vi "MainRunExp.vi"() -> ()   [LabVIEW 2019, in "MotorPID.lvlib"]
uses:
  MotorPID.lvlib
  RunState.ctl
  KNRm_ReMi_OS5.lvlibp/KNRm_ReMi_Toolkit/IO/LowLevel/IO_Channel_DIO.ctl
  <vilib>/Platform/TimedLoop/XDataNode/timing_clust.ctl
  <vilib>/Platform/TimedLoop/XDataNode/nitl_modes.ctl
  <vilib>/Platform/TimedLoop/XDataNode/wakeup.ctl
  <vilib>/addons/control/pid/pid.llb/PID (DBL).vi
  <vilib>/Platform/TimedLoop/XDataNode/XDataNode.xnode
  <vilib>/addons/control/pid/NI_PID_pid.lvlib
  <vilib>/Platform/TimedLoop/XDataNode/XDNodeRunTimeDep.lvlib
  <vilib>/ptbypt/NI_PtbyPt.lvlib
  KNRm_ReMi_OS5.lvlibp
panel:
  out "x .or. y? 2":bool
  out "x .or. y?":bool
  out "Boolean":bool
  out "State":u16(ring) items=["StickReset", "MotorReset", "MotorHome", "RunUp", "Runing", "Exit"]
  out "Waveform Chart":T1(graph)
  in  "Setpoint(deg)":dbl(knob) scale=80.0..-80.0
  out "error out":errorcluster
  out "Position(deg)":dbl(knob) scale=80.0..-80.0
  in  "Reset":bool
  in  "Stop Button":bool
  out "MotorResetPOS":dbl[](array[numeric])
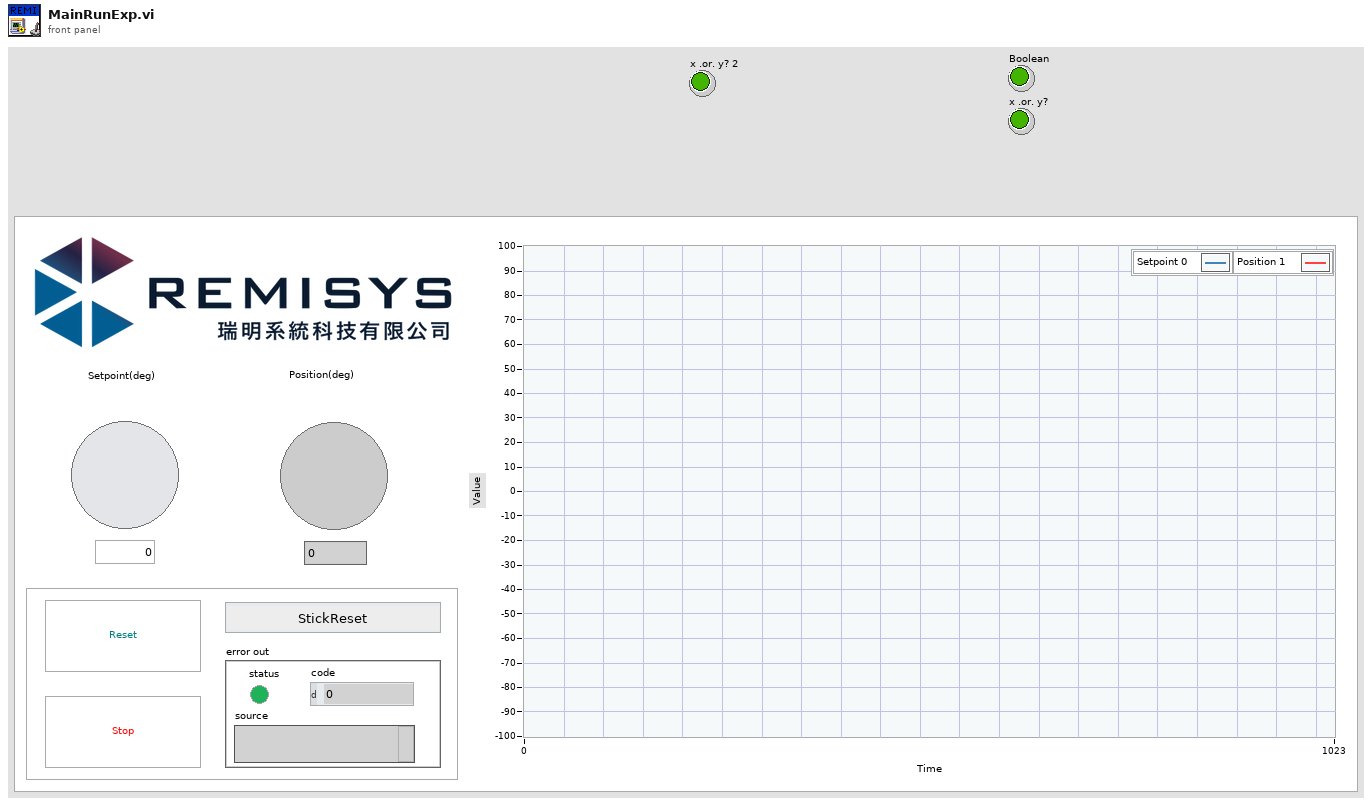
[diagram p1: front panel]
types:
  T1 = cluster{"Setpoint(deg)":dbl, "PresentPOS(deg)":dbl}
  T2 = typedef "MotorPID.lvlib/RunState.ctl" = enum16{"StickReset", "MotorReset", "MotorHome", "RunUp", "Runing", "Exit"}
  T3 = typedef "KNRm_ReMi_OS5.lvlibp/IO_Channel_DIO.ctl" = enum16{"B/DIO1 (M1)", "A/DIO8 (M2)", "B/DIO7 (M3)", "A/DIO3 (M4)", "A/DIO14 (RC1_0)", "A/DIO15 (RC1_1)"}
  T4 = typedef "XDNodeRunTimeDep.lvlib/timing_clust.ctl" = cluster{"Expected End [f-1]":u64, "Actual End [f-1]":u64, "Finished Late? [f-1]":bool, "Expected End [i-1]":u64, "Actual End [i-1]":u64, "Finished Late? [i-1]":bool, "Expected Start [i]":u64, "Actual Start [i]":u64, "Expected Start [f]":u64, "Actual Start [f]":u64, "Source Name":string, "Structure Name":string, "Period":i64, "Deadline":i64, "Offset":i64, "Start":i64, "Priority":i32, "Timeout":i32, "Mode":T5, "Wakeup Reason":T6, "Error":errorcluster, "Source Type":string, "Secondary Source Type":string, "Global End Time":u64, "Global Start Time":u64, "Frame Duration":u64, "Iteration Duration":u64, "Assigned CPU":i32, "I/O Scan Engine Mode":u32}
  T5 = typedef "XDNodeRunTimeDep.lvlib/nitl_modes.ctl" = enum32{"No Change", "Process missed periods, maintain original phase", "Discard missed periods, maintain original phase", "Process missed periods, ignore original phase", "Discard missed periods, ignore original phase"}
  T6 = typedef "XDNodeRunTimeDep.lvlib/wakeup.ctl" = enum32{"Normal", "Aborted", "Asynchronous wakeup", "Timing source error", "Timed loop error", "Timeout"}
  T7 = cluster{"proportional gain (Kc)":dbl, "integral time (Ti, min)":dbl, "derivative time (Td, min)":dbl}
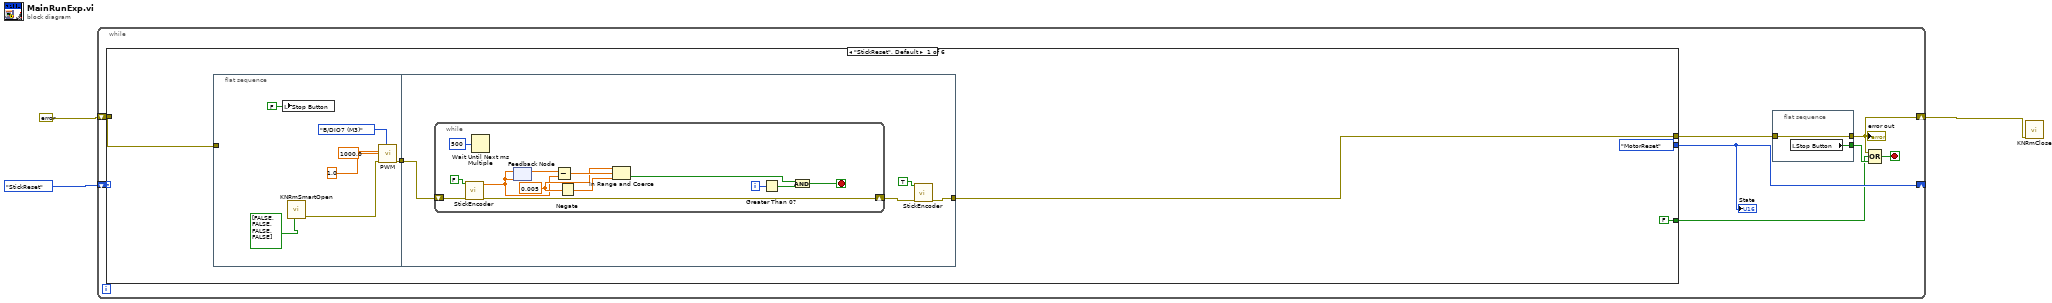
[diagram p0: block diagram]
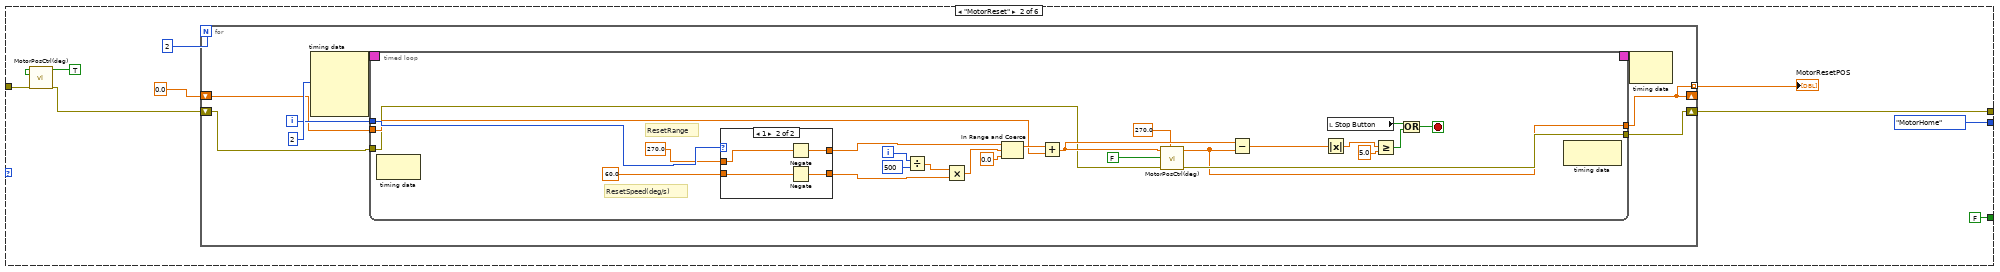
[diagram p2: hidden frame]
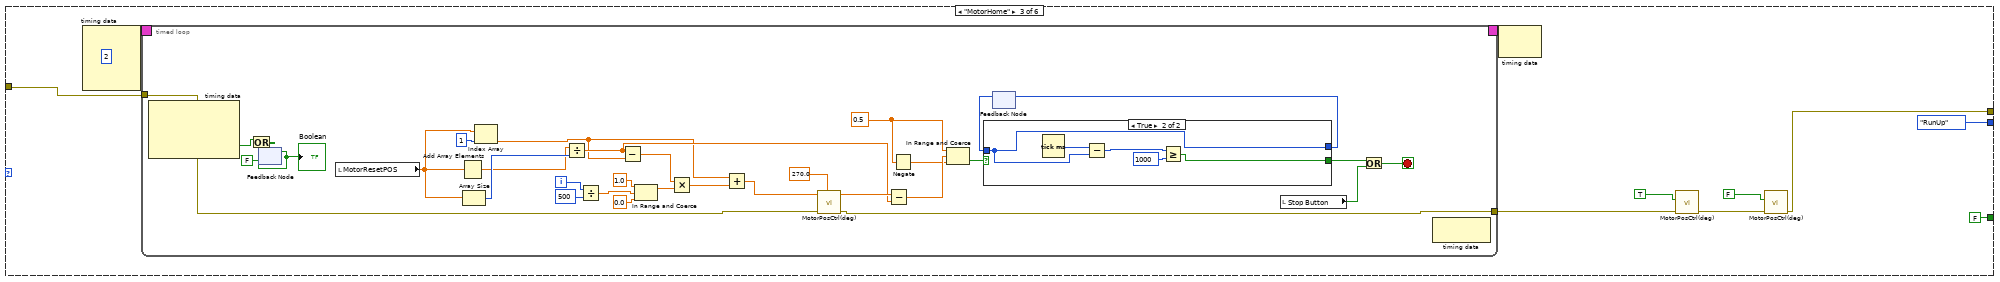
[diagram p4: hidden frame]
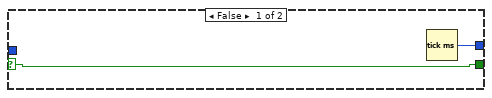
[diagram p5: hidden frame]
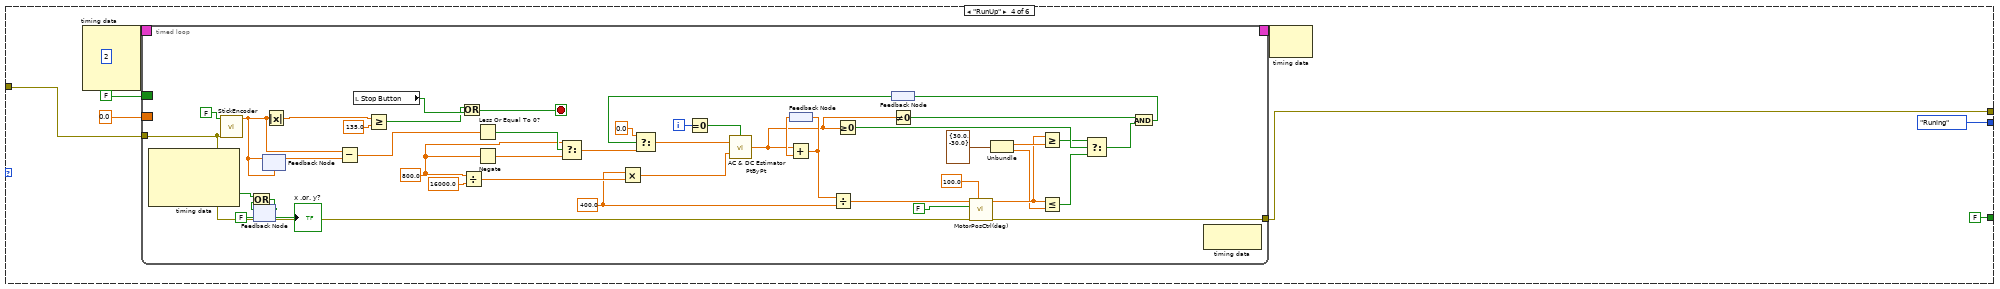
[diagram p6: hidden frame]
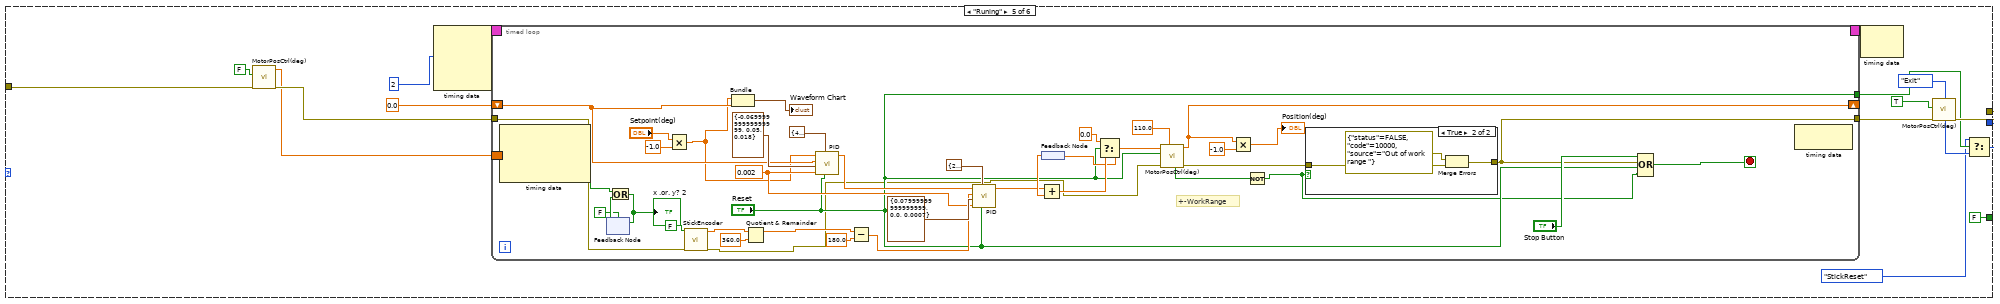
[diagram p7: hidden frame]
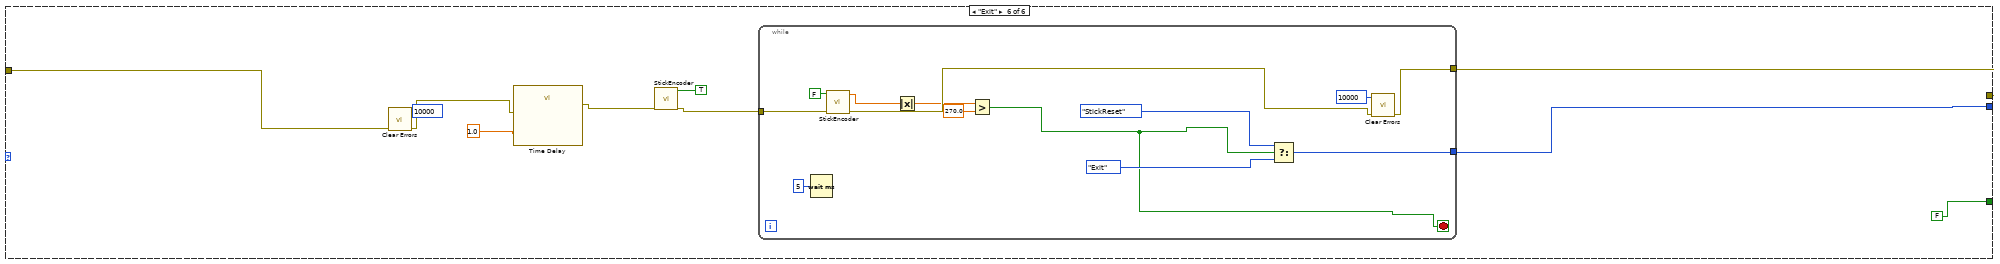
[diagram p9: hidden frame]
diagram:
  n1 = while {
    shift-right: [w6] -> _
    shift-left: RunState."StickReset" -> [w11]
    shift-right: [w5] -> w1
    shift-left: errorcluster {"status"=FALSE, "code"=0, "source"=""} ("error in (no error)") -> [w10]
    stop <- w9 stop-if-true
    n2 = case shown="\"StickReset\", Default" w11 {
      tunnel: w10 -> [w16 w45 w103 w158 w224 w281]
      tunnel: [w17 w51 w97 w156 w218 w283] -> w8
      tunnel: [RunState."MotorReset" RunState."MotorHome" RunState."RunUp" RunState."Runing" w214 w284] -> w6
      tunnel: [FALSE FALSE FALSE FALSE FALSE FALSE] -> w4
      frame "StickReset", Default {
        n3 = flat-sequence {
          tunnel: w16 -> [_]
          tunnel: [w19] -> w15
          tunnel: [w27] -> w17
          tunnel: w15 -> [w26]
          frame #0 {
            n4 = local write "Stop Button"(FALSE ("Stop Button")) -> ()
            n5 = call "KNRmSmartOpen.vi"("SpeedMode"=bool[] [FALSE, FALSE, FALSE, FALSE]) -> ("error out"=w22:errorcluster)  [unwired: 8 in, 2 out]
            n6 = call "PWM.vi"("IO_Chanel"=IO_Channel_DIO."B/DIO7 (M3)", "error in"=w22, "DutyCycle"=1.0, "Frequency(Hz)"=1000.0) -> ("error out"=w19:errorcluster)  [unwired: 7 in]
          }
          frame #1 {
            n7 = while {
              shift-right: [w42] -> w29
              shift-left: w26 -> [w41]
              i -> [w35]
              stop <- w32 stop-if-true
              w37 = 0.005 ("upper limit")
              n8 = call "StickEncoder.vi"("error in (no error)"=w41, "Reset Counter"=FALSE) -> ("error out"=w42:errorcluster, "PresentPOS(deg)"=w30:dbl)  [unwired: 8 in]
              n9 = Wait Until Next ms Multiple(millisecond multiple=u32 500) -> ()  [unwired: 1 out]
              n10 = feedback-in #1(w30) -> ()
              n11 = feedback #1(w30) -> (w39:dbl)
              n12 = Subtract(x=w39, y=w30) -> (x-y=w38:dbl)
              n13 = Negate(x=w37) -> (-x=w36:dbl)
              n14 = In Range and Coerce(upper limit=w37, x=w38, lower limit=w36) -> (In Range?=w34:bool)  [unwired: 1 out]
              n15 = Greater Than 0?(x=w35) -> (x > 0?=w33:bool)
              n16 = And(x=w34, y=w33) -> (x .and. y?=w32:bool)
            }
            n17 = call "StickEncoder.vi"("error in (no error)"=w29, "Reset Counter"=TRUE) -> ("error out"=w27:errorcluster)  [unwired: 8 in, 1 out]
          }
        }
      }
      frame "MotorReset" {
        n18 = call "MotorPosCtrl(deg).vi"("error in (no error)"=w45, "Reset Button"=TRUE) -> ("error out"=w46:errorcluster)  [unwired: 7 in, 2 out]
        n19 = for {
          N: 2 -> [_]
          shift-right: [w56] -> w51
          shift-left: w46 -> [w55]
          shift-right: [w52] -> _
          shift-left: 0.0 ("PresentPOS(deg)") -> [w53]
          tunnel: [w52] -> w48 mode=indexing
          i -> [w54]
          n20 = node-c288(i64 2 ("Period")) -> (w59:T4)  [unwired: 3 in]
          n21 = timed-loop {
            timing: w59 -> [_]
            timing-out: [_] -> w58
            tunnel: w55 -> [w60]
            tunnel: [w83] -> w56
            tunnel: w54 -> [w78]
            tunnel: [w66] -> w52
            tunnel: w53 -> [w75]
            i -> [w82]
            stop <- w70 stop-if-true
            # "ResetRange"
            # "ResetSpeed(deg/s)"
            n22 = node-c288() -> ()  [unwired: 1 in, 1 out]
            n23 = case shown="1" w78 {
              tunnel: [w85 w88] -> w77
              tunnel: [w84 w86] -> w73
              tunnel: 270.0 ("Target(deg)") -> [w85 w89]
              tunnel: 60.0 ("y") -> [w84 w87]
              frame 0, Default {
              }
              frame 1 {
                n24 = Negate(x=w89) -> (-x=w88:dbl)
                n25 = Negate(x=w87) -> (-x=w86:dbl)
              }
            }
            n26 = Divide(x=w82, y=500) -> (x/y=w81:dbl)
            n27 = Multiply(x=w81, y=w73) -> (x*y=w80:dbl)
            n28 = In Range and Coerce(upper limit=w77, x=w80, lower limit=0.0) -> (coerced(x)=w76:dbl)  [unwired: 1 out]
            n29 = Add(x=w76, y=w75) -> (x+y=w67:dbl)
            n30 = call "MotorPosCtrl(deg).vi"("WorkRange"=270.0, "error in (no error)"=w60, "Reset Button"=FALSE, "Target(deg)"=w67) -> ("error out"=w83:errorcluster, "PresentPOS(deg)"=w66:dbl)  [unwired: 5 in, 1 out]
            n31 = Subtract(x=w67, y=w66) -> (x-y=w64:dbl)
            n32 = Absolute Value(x=w64) -> (abs(x)=w63:dbl)
            n33 = local read "Stop Button"() -> (w69:bool)
            n34 = Greater Or Equal?(x=w63, y=5.0) -> (x >= y?=w62:bool)
            n35 = Or(x=w69, y=w62) -> (x .or. y?=w70:bool)
            n36 = node-c288() -> ()  [unwired: 1 in, 1 out]
          }
          n37 = node-c288(w58) -> ()  [unwired: 1 out]
        }
        "MotorResetPOS" <- w48
      }
      frame "MotorHome" {
        n38 = node-c288(i64 2 ("Period")) -> (w105:T4)  [unwired: 3 in]
        n39 = timed-loop {
          timing: w105 -> [_]
          timing-out: [_] -> w104
          tunnel: w103 -> [w138]
          tunnel: [w132] -> w101
          i -> [w126]
          stop <- w112 stop-if-true
          w134 = 0.5
          n40 = node-c288() -> (w110:bool)  [unwired: 1 in, 3 out]
          n41 = feedback #2(FALSE) -> (w108:bool)
          "Boolean" <- w108
          n42 = Or(x=w110, y=w108) -> (x .or. y?=w109:bool)
          n43 = feedback-in #2(w109) -> ()
          n44 = local read "MotorResetPOS"() -> (w121:dbl[])
          n45 = Add Array Elements(numeric array=w121) -> (sum=w120:dbl)
          n46 = Array Size(array=w121) -> (size(s)=w137:i32)
          n47 = Index Array(array=w121, index=1) -> (element=w115:dbl)
          n48 = Divide(x=w120, y=w137) -> (x/y=w117:dbl)
          n49 = Divide(x=w126, y=500) -> (x/y=w124:dbl)
          n50 = Subtract(x=w117, y=w115) -> (x-y=w116:dbl)
          n51 = In Range and Coerce(upper limit=1.0, x=w124, lower limit=0.0) -> (coerced(x)=w119:dbl)  [unwired: 1 out]
          n52 = Multiply(x=w116, y=w119) -> (x*y=w118:dbl)
          n53 = Add(x=w115, y=w118) -> (x+y=w114:dbl)
          n54 = call "MotorPosCtrl(deg).vi"("WorkRange"=270.0, "error in (no error)"=w138, "Target(deg)"=w114) -> ("error out"=w132:errorcluster, "PresentPOS(deg)"=w136:dbl)  [unwired: 6 in, 1 out]
          n55 = Subtract(x=w136, y=w117) -> (x-y=w135:dbl)
          n56 = Negate(x=w134) -> (-x=w133:dbl)
          n57 = In Range and Coerce(upper limit=w134, x=w135, lower limit=w133) -> (In Range?=w127:bool)  [unwired: 1 out]
          n58 = feedback #3() -> (w130:u32)  [unwired: 1 in]
          n59 = case shown="True" w127 {
            selector: w127 -> [w139 _]
            tunnel: [w140 w141] -> w131
            tunnel: w130 -> [_ w141]
            tunnel: [w139 w142] -> w128
            frame False {
              n60 = Tick Count (ms)() -> (millisecond timer value=w140:u32)
            }
            frame True {
              n61 = Tick Count (ms)() -> (millisecond timer value=w145:u32)
              n62 = Subtract(x=w145, y=w141) -> (x-y=w144:u32)
              n63 = Greater Or Equal?(x=w144, y=u32 1000) -> (x >= y?=w142:bool)
            }
          }
          n64 = feedback-in #3(w131) -> ()
          n65 = local read "Stop Button"() -> (w129:bool)
          n66 = Or(x=w128, y=w129) -> (x .or. y?=w112:bool)
          n67 = node-c288() -> ()  [unwired: 1 in, 1 out]
        }
        n68 = node-c288(w104) -> ()  [unwired: 1 out]
        n69 = call "MotorPosCtrl(deg).vi"("error in (no error)"=w101, "Reset Button"=TRUE) -> ("error out"=w98:errorcluster)  [unwired: 7 in, 2 out]
        n70 = call "MotorPosCtrl(deg).vi"("error in (no error)"=w98, "Reset Button"=FALSE) -> ("error out"=w97:errorcluster)  [unwired: 7 in, 2 out]
      }
      frame "RunUp" {
        n71 = node-c288(i64 2 ("Period")) -> (w161:T4)  [unwired: 3 in]
        n72 = timed-loop {
          timing: w161 -> [_]
          timing-out: [_] -> w160
          tunnel: w158 -> [w203]
          tunnel: [w198] -> w156
          border: 0.0 ("PresentPOS(deg)") -> [_]
          border: FALSE -> [_]
          i -> [w205]
          stop <- w195 stop-if-true
          w191 = 800.0 ("MaxSpeed(deg/s)")
          w181 = 400.0 ("x")
          n73 = node-c288() -> (w165:bool)  [unwired: 1 in, 3 out]
          n74 = call "StickEncoder.vi"("error in (no error)"=w203, "Reset Counter"=FALSE) -> ("PresentPOS(deg)"=w168:dbl)  [unwired: 8 in, 1 out]
          n75 = feedback #4(FALSE) -> (w163:bool)
          n76 = Or(x=w165, y=w163) -> (x .or. y?=w164:bool)
          "x .or. y?" <- w164
          n77 = feedback-in #4(w164) -> ()
          n78 = feedback-in #5(w168) -> ()
          n79 = feedback #5(w168) -> (w201:dbl)
          n80 = Absolute Value(x=w168) -> (abs(x)=w200:dbl)
          n81 = Subtract(x=w168, y=w201) -> (x-y=w194:dbl)
          n82 = local read "Stop Button"() -> (w197:bool)
          n83 = Greater Or Equal?(x=w200, y=135.0) -> (x >= y?=w196:bool)
          n84 = Or(x=w196, y=w197) -> (x .or. y?=w195:bool)
          n85 = Divide(x=w191, y=16000.0 ("Acc(deg/ss)")) -> (x/y=w190:dbl)
          n86 = Less Or Equal To 0?(x=w194) -> (x <= 0?=w193:bool)
          n87 = Negate(x=w191) -> (-x=w192:dbl)
          n88 = Select(t=w191, s=w193, f=w192) -> (s? t:f=w185:dbl)
          n89 = Multiply(x=w181, y=w190) -> (x*y=w167:dbl)
          n90 = Equal To 0?(x=w205) -> (x = 0?=w204:bool)
          n91 = feedback #6() -> (w188:dbl)
          n92 = feedback #7() -> (w186:bool)
          n93 = Select(t=0.0, s=w186, f=w185) -> (s? t:f=w183:dbl)
          n94 = call <vilib>:"AC & DC Estimator PtByPt.vi"("signal"=w183, "sample length"=w167, "initialize"=w204) -> ("DC estimate (V)"=w172:dbl)  [unwired: 2 out]
          n95 = Add(x=w172, y=w188) -> (x+y=w182:dbl)
          n96 = feedback-in #6(w182) -> ()
          n97 = Divide(x=w182, y=w181) -> (x/y=w180:dbl)
          n98 = Greater Or Equal To 0?(x=w172) -> (x >= 0?=w178:bool)
          n99 = Not Equal To 0?(x=w172) -> (x != 0?=w171:bool)
          n100 = call "MotorPosCtrl(deg).vi"("WorkRange"=100.0, "error in (no error)"=w203, "Reset Button"=FALSE, "Target(deg)"=w180) -> ("error out"=w198:errorcluster, "PresentPOS(deg)"=w176:dbl)  [unwired: 5 in, 1 out]
          n101 = Unbundle(cluster{"UpLimit":dbl, "DownLimit":dbl} {"UpLimit"=30.0, "DownLimit"=-30.0} ("RunUpLimuit")) -> ("UpLimit"=w177:dbl, "DownLimit"=w175:dbl)
          n102 = Greater Or Equal?(x=w176, y=w177) -> (x >= y?=w174:bool)
          n103 = Less Or Equal?(x=w176, y=w175) -> (x <= y?=w173:bool)
          n104 = Select(t=w174, s=w178, f=w173) -> (s? t:f=w170:bool)
          n105 = And(x=w171, y=w170) -> (x .and. y?=w169:bool)
          n106 = feedback-in #7(w169) -> ()
          n107 = node-c288() -> ()  [unwired: 1 in, 1 out]
        }
        n108 = node-c288(w160) -> ()  [unwired: 1 out]
      }
      frame "Runing" {
        n109 = call "MotorPosCtrl(deg).vi"("error in (no error)"=w224, "Reset Button"=FALSE) -> ("error out"=w223:errorcluster, "PresentPOS(deg)"=w221:dbl)  [unwired: 7 in, 1 out]
        n110 = node-c288(i64 2 ("Period")) -> (w228:T4)  [unwired: 3 in]
        n111 = timed-loop "Timed Loop" {
          tunnel: [w244] -> w220
          timing: w228 -> [_]
          timing-out: [_] -> w227
          border: w221 -> [_]
          shift-right: [w231] -> _
          shift-left: 0.0 -> [w242]
          tunnel: w223 -> [w253]
          tunnel: ["Reset"] -> w217
          stop <- w245 stop-if-true
          w259 = 0.002 ("dt (s)")
          # "+-WorkRange"
          n112 = node-c288() -> (w237:bool)  [unwired: 1 in, 3 out]
          n113 = feedback #8(FALSE) -> (w239:bool)
          n114 = Or(x=w237, y=w239) -> (x .or. y?=w240:bool)
          "x .or. y? 2" <- w240
          n115 = feedback-in #8(w240) -> ()
          n116 = Multiply(x="Setpoint(deg)", y=-1.0) -> (x*y=w234:dbl)
          n117 = call "StickEncoder.vi"("error in (no error)"=w253, "Reset Counter"=FALSE) -> ("error out"=w236:errorcluster, "PresentPOS(deg)"=w251:dbl)  [unwired: 8 in]
          n118 = Bundle(w234, w242) -> (→"Waveform Chart":cluster{dbl, dbl})  [unwired: 1 in]
          n119 = Quotient & Remainder(x=w251, y=360.0) -> (x-y*floor(x/y)=w250:dbl)  [unwired: 1 out]
          n120 = call-poly <vilib>:"PID.vi"("reinitialize? (F)"="Reset", "output range"=cluster{"output high":dbl, "output low":dbl} {"output high"=45.0, "output low"=-45.0}, "dt (s)"=w259, "PID gains"=T7 {"proportional gain (Kc)"=-0.06999999999999999, "integral time (Ti, min)"=0.05, "derivative time (Td, min)"=0.018} ("PID gains 2"), "process variable"=w242, "setpoint"=w234) -> ("output"=w254:dbl)  [unwired: 4 in, 1 out]
          n121 = Subtract(x=w250, y=180.0) -> (x-y=w258:dbl)
          n122 = call-poly <vilib>:"PID.vi"("reinitialize? (F)"="Reset", "output range"=cluster{"output high":dbl, "output low":dbl} {"output high"=2.0, "output low"=-2.0}, "dt (s)"=w259, "PID gains"=T7 {"proportional gain (Kc)"=0.07999999999999999, "integral time (Ti, min)"=0.0, "derivative time (Td, min)"=0.0007}, "process variable"=w258, "setpoint"=w254) -> ("output"=w256:dbl)  [unwired: 4 in, 1 out]
          n123 = feedback #9() -> (w264:dbl)
          n124 = Add(x=w256, y=w264) -> (x+y=w263:dbl)
          n125 = Select(t=0.0, s="Reset", f=w263) -> (s? t:f=w261:dbl)
          n126 = feedback-in #9(w261) -> ()
          n127 = call "MotorPosCtrl(deg).vi"("WorkRange"=110.0, "error in (no error)"=w236, "Reset Button"="Reset", "Target(deg)"=w261) -> ("error out"=w247:errorcluster, "PresentPOS(deg)"=w231:dbl, "In Range?"=w248:bool)  [unwired: 5 in]
          n128 = Multiply(x=w231, y=-1.0) -> (x*y=→"Position(deg)":dbl)
          n129 = Not(x=w248) -> (.not. x?=w229:bool)
          n130 = case shown="True" w229 {
            tunnel: w247 -> [w268 w271]
            tunnel: [w268 w269] -> w244
            frame False {
            }
            frame True {
              n131 = Merge Errors(errorcluster {"status"=FALSE, "code"=10000, "source"="Out of work range "} ("error in (no error)"), w271) -> (w269:errorcluster)
            }
          }
          n132 = Compound Arithmetic op=OR("Stop Button", w244, "Reset", w229) -> (w245:bool)
          n133 = node-c288() -> ()  [unwired: 1 in, 1 out]
        }
        n134 = node-c288(w227) -> ()  [unwired: 1 out]
        n135 = call "MotorPosCtrl(deg).vi"("error in (no error)"=w220, "Reset Button"=TRUE) -> ("error out"=w218:errorcluster)  [unwired: 7 in, 2 out]
        n136 = Select(t=RunState."StickReset", s=w217, f=RunState."Exit") -> (s? t:f=w214:T2)
      }
      frame "Exit" {
        n137 = call <vilib>:"Clear Errors.vi"("error in (no error)"=w281, "specific error code to clear (0: all)"=10000) -> ("error out"=w280:errorcluster)  [unwired: 4 in, 1 out]
        n138 = call "Time Delay"("error in (no error)"=w280, "Delay Time (s)"=1.0) -> ("error out"=w286:errorcluster)  [unwired: 9 in]
        n139 = call "StickEncoder.vi"("error in (no error)"=w286, "Reset Counter"=TRUE) -> ("error out"=w285:errorcluster)  [unwired: 8 in, 1 out]
        n140 = while {
          tunnel: w285 -> [w301]
          tunnel: [w295] -> w284
          tunnel: [w291] -> w283
          stop <- w290 stop-if-true
          n141 = Wait (ms)(milliseconds to wait=u32 5) -> ()  [unwired: 1 out]
          n142 = call "StickEncoder.vi"("error in (no error)"=w301, "Reset Counter"=FALSE) -> ("error out"=w292:errorcluster, "PresentPOS(deg)"=w298:dbl)  [unwired: 8 in]
          n143 = Absolute Value(x=w298) -> (abs(x)=w289:dbl)
          n144 = Greater?(x=w289, y=270.0) -> (0:w290:bool)
          n145 = Select(t=RunState."StickReset", s=w290, f=RunState."Exit") -> (s? t:f=w295:T2)
          n146 = call <vilib>:"Clear Errors.vi"("error in (no error)"=w292, "specific error code to clear (0: all)"=10000) -> ("error out"=w291:errorcluster)  [unwired: 4 in, 1 out]
        }
      }
    }
    "State" <- w6
    n147 = flat-sequence {
      tunnel: w8 -> [w12]
      tunnel: [w13] -> w7
      tunnel: [w12] -> w5
      frame #0 {
        n148 = local read "Stop Button"() -> (w13:bool)
      }
    }
    n149 = Compound Arithmetic op=OR(w5, w4, w7) -> (w9:bool)
    "error out" <- w5
  }
  n150 = call "KNRmClose.vi"("error in"=w1) -> ()  [unwired: 10 in, 1 out]
